vi "Test_Copy_To_Raw_Memory_ARGB.vi"(8 "error in (no error)":errorcluster, 11 "Test Case In":refnum<class "Image.lvclass">) -> (0 "error out":errorcluster, 3 "Test Case Out":refnum<class "Image.lvclass">)   [LabVIEW 2020, in "g_ar_toolkit.test.lvlib" / "Image.lvclass"]
uses:
  Image.lvclass
  Image.lvclass/Image.ctl
  g_ar_toolkit.image/Image Size (Fixed).ctl
  g_ar_toolkit.image/g_ar_toolkit.image.lvlib
  g_ar_toolkit.image/Raw Memory Information Dimension.ctl
  g_ar_toolkit.image/Raw Memory Information.ctl
  g_ar_toolkit.image/CreateEmptyImageARGB.vi
  4993e8ee-a06a-463a-9684-69129f64d5ce.vi
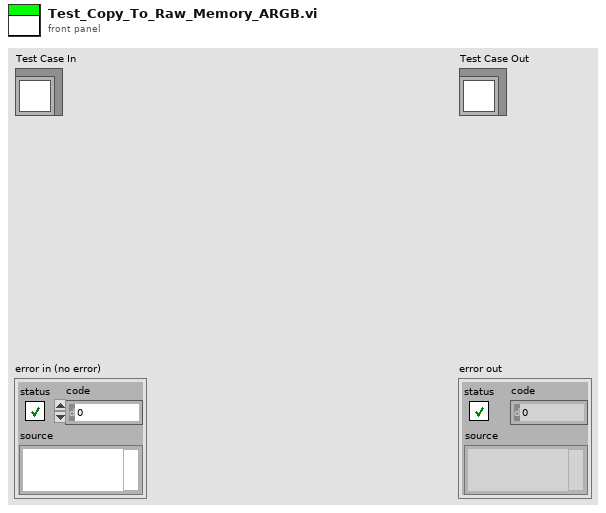
[diagram p1: front panel]
types:
  T1 = typedef "g_ar_toolkit.image.lvlib/Image Size (Fixed).ctl" = cluster{"Width":u16, "Height":u16}
  T2 = typedef "imagedata.ctl" = cluster{"image type":i32, "image depth":i32, "image":u8[], "mask":u8[], "colors":u32[], "Rectangle":cluster{"left":i16, "top":i16, "right":i16, "bottom":i16}}
  T3 = typedef "g_ar_toolkit.image.lvlib/Raw Memory Information.ctl" = cluster{"Memory Address":u64, "Dimension 0":T4, "Dimension 1":T4}
  T4 = typedef "g_ar_toolkit.image.lvlib/Raw Memory Information Dimension.ctl" = cluster{"Size":u16, "Stride":u32}
  T5 = cluster{"pointer":u64, "size_0":u32, "stride_0":i32, "size_1":u32, "stride_1":i32, "element size":u32, "subarray?":bool}
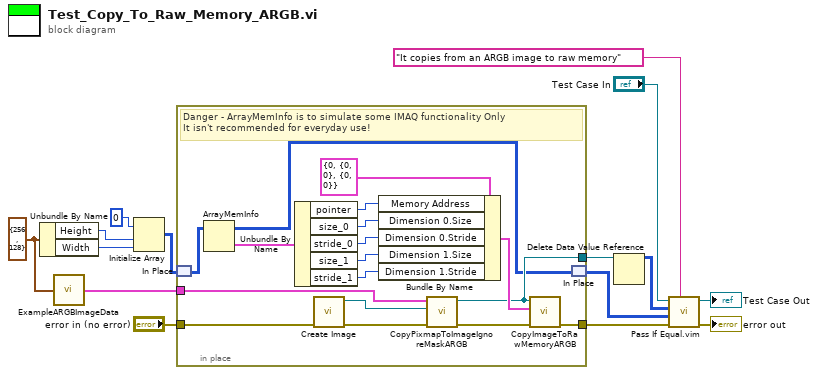
[diagram p0: block diagram]
diagram:
  w11 = T1 {"Width"=256, "Height"=128} ("Image Size")
  n1 = Unbundle By Name(w11) -> ("Height"=w9:u16, "Width"=w8:u16)
  n2 = call "ExampleARGBImageData.vi"("Image Size"=w11) -> ("RGB Image Data"=w10:T2)
  n3 = Initialize Array(u32 0, w9, w8) -> (w3:u32[][])
  n4 = in-place {
    in-place-border: w10 -> [w32]
    in-place-border: "error in (no error)" -> [w22]
    in-place-border: [w21] -> w6
    in-place-border: [w18] -> w4
    # "Danger - ArrayMemInfo is to simulate some IMAQ functionality Only\nIt isn't recommended for everyday use!"
    n5 = in-place-match #1(w3) -> (w16:u32[][])
    n6 = ArrayMemInfo(3:w16) -> (0:w30:T5, 1:w17:u32[][])
    n7 = Unbundle By Name(w30) -> ("pointer"=w28:u64, "size_0"=w26:u32, "stride_0"=w25:i32, "size_1"=w23:u32, "stride_1"=w24:i32)
    n8 = call-poly "Create Image.vi"("error in (no error)"=w22) -> ("error out"=w19:errorcluster, "New ARGB Image"=w31:refnum<data-value>)  [unwired: 9 in]
    n9 = Bundle By Name(cluster=T3 {"Memory Address"=0, "Dimension 0"={"Size"=0, "Stride"=0}, "Dimension 1"={"Size"=0, "Stride"=0}} ("Destination"), "Memory Address"=w28, "Dimension 0.Size"=w26, "Dimension 0.Stride"=w25, "Dimension 1.Size"=w23, "Dimension 1.Stride"=w24) -> (w27:T3)
    n10 = call "CopyPixmapToImageIgnoreMaskARGB.vi"("error in (no error)"=w19, "ARGB Image Destination"=w31, "Pixmap Image Data"=w32) -> ("error out"=w20:errorcluster, "ARGB Image Destination (duplicate)"=w21:refnum<data-value>)  [unwired: 7 in]
    n11 = call "CopyImageToRawMemoryARGB.vi"("error in (no error)"=w20, "Destination"=w27, "ARGB Image Source"=w21) -> ("error out"=w18:errorcluster)  [unwired: 7 in, 1 out]
    n12 = in-place-match #1(w17) -> (w2:u32[][])
  }
  n13 = Delete Data Value Reference(data value reference=w6) -> (data value=w5:u32[][])  [unwired: 1 in, 1 out]
  n14 = call "Pass If Equal.vim"("Description"="It copies from an ARGB image to raw memory", "error in (no error)"=w4, "Actual"=w2, "Expected"=w5, "LUnit Test Case In"="Test Case In") -> ("error out"=→"error out":errorcluster, "LUnit Test Case Out"=→"Test Case Out":refnum<class "Image.lvclass">)  [unwired: 5 in]
